vi "Build Dictionary.vi"(8 "error in (no error)":errorcluster, 11 "Response Headers in":refnum<class "Response Headers.lvclass">) -> (0 "error out":errorcluster, 3 "Response Headers out":refnum<class "Response Headers.lvclass">)   [LabVIEW 2018, in "REST Client_JKI.lvlib" / "Response Headers.lvclass"]
uses:
  Response Headers.lvclass
  Response Headers.lvclass/Response Headers.ctl
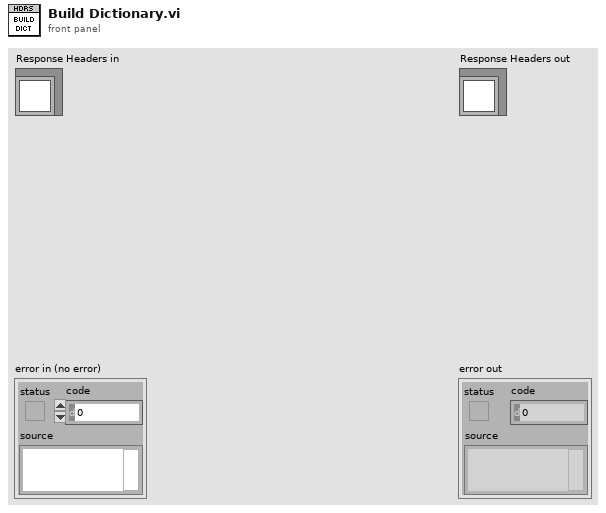
[diagram p1: front panel]
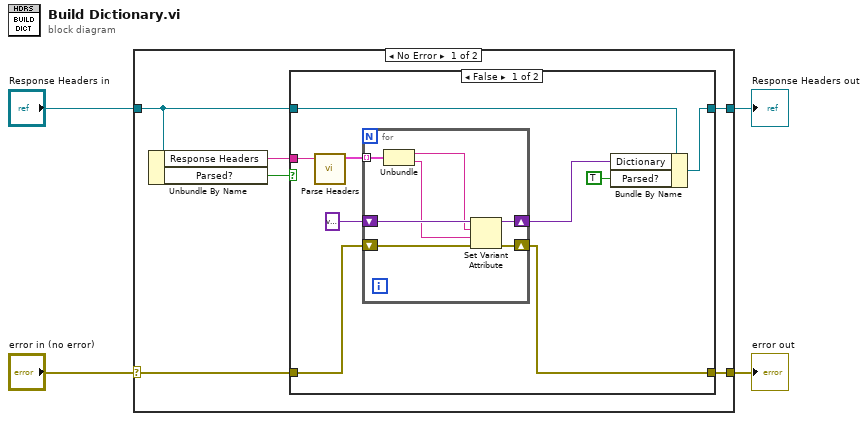
[diagram p0: block diagram]
diagram:
  n1 = case shown="No Error" "error in (no error)" {
    selector: "error in (no error)" -> [w7 w30]
    tunnel: [w6 w30] -> w3
    tunnel: [w8 w29] -> w1
    tunnel: "Response Headers in" -> [w9 w29]
    frame No Error {
      n2 = Unbundle By Name(w9) -> ("Response Headers"=w10:string, "Parsed?"=w5:bool)
      n3 = case shown="False" w5 {
        tunnel: w10 -> [w19 _]
        tunnel: w9 -> [w17 w28]
        tunnel: [w16 w28] -> w8
        tunnel: w7 -> [w13 w27]
        tunnel: [w12 w27] -> w6
        frame False {
          n4 = call "Parse Headers.vi"("HTTP Headers"=w19) -> ("Response Headers"=w18:cluster{"header":string, "value":string}[])  [unwired: 10 in]
          n5 = for {
            tunnel: w18 -> [w26] mode=indexing
            shift-right: [w25] -> w11
            shift-left: variant ("variant") -> [w24]
            shift-right: [w20] -> w12
            shift-left: w13 -> [w21]
            n6 = Unbundle(w26) -> ("header"=w23:string, "value"=w22:string)
            n7 = Set Variant Attribute(Variant=w24, name=w23, value=w22, error in=w21) -> (Variant out=w25:variant, error out=w20:errorcluster)  [unwired: 1 out]
          }
          n8 = Bundle By Name(cluster=w17, "Dictionary"=w11, "Parsed?"=TRUE) -> (w16:refnum<class "Response Headers.lvclass">)
        }
        frame True {
        }
      }
    }
    frame Error {
    }
  }
  "error out" <- w3
  "Response Headers out" <- w1
